vi "Read.vi"(8 "error in (no error)":errorcluster, 9 "Sample Rate [Hz]":dbl=1000.0 min=1000.0 max=8000000.0, 10 "Number of Samples":u32=1000, 11 "DI (N Samples) Ref In":T1) -> (0 "error out":errorcluster, 2 "Values":bool[][](array[boolean]), 3 "DI (N Samples) Ref Out":T1)   [LabVIEW 2021, in "DI Block.lvlib"]
doc: "Reads values from one or more digital input channels. Use this VI to read multiple samples for each channel at one time."
uses:
  <vilib>/myRIO/Instrument Drivers/Onboard IO/DI Block/DI Block.lvlib
  <vilib>/myRIO/Instrument Drivers/Onboard IO/DI Block/typedefs/DI Block Reference.ctl
  <vilib>/myRIO/Common/Instrument Driver Framework/Utilities/typedefs/myRIO Generic Hardware Reference.ctl
  <vilib>/myRIO/Common/Instrument Driver Framework/Utilities/typedefs/Hardware Version Enum.ctl
  <vilib>/myRIO/Common/Instrument Driver Framework/Utilities/typedefs/myRIO v1.0 Reference.ctl
  <vilib>/myRIO/Common/Instrument Driver Framework/Utilities/typedefs/Generic FPGA Reference.ctl
  <vilib>/myRIO/Common/Instrument Driver Framework/myRIO v1.0/DI Block/typedefs/DI Block Channels List.ctl
  <vilib>/myRIO/Common/Instrument Driver Framework/myRIO v1.0/DI Block/typedefs/DI Block Channels Enum.ctl
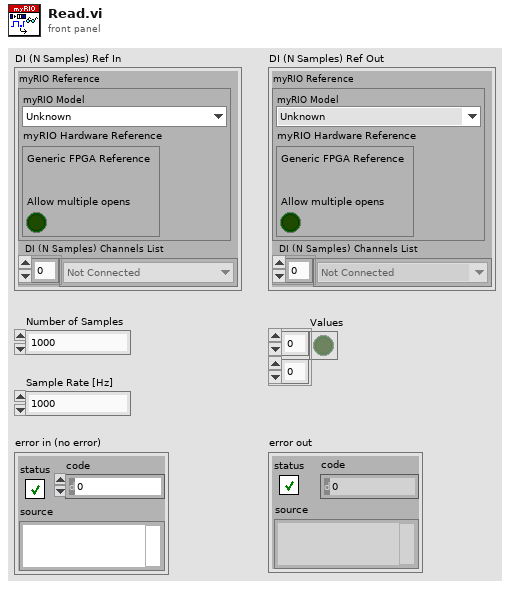
[diagram p1: front panel]
types:
  T1 = typedef "DI Block.lvlib/DI Block Reference.ctl" = cluster{"myRIO Reference":T2, "DI (N Samples) Channels List":T6}
  T2 = typedef "myRIO Generic Hardware Reference.ctl" = cluster{"myRIO Model":T3, "myRIO Hardware Reference":T4}
  T3 = typedef "Hardware Version Enum.ctl" = enum16{"Unknown", "myRIO-1900", "myRIO-1950", "roboRIO", "NI ELVIS RIO CM", "ELVIS III"}
  T4 = typedef "myRIO v1.0 Reference.ctl" = cluster{"Generic FPGA Reference":T5, "Allow multiple opens":bool}
  T5 = typedef "Generic FPGA Reference.ctl" = refnum<k20>
  T6 = typedef "DI Block Channels List.ctl" = T7[]
  T7 = typedef "DI Block Channels Enum.ctl" = enum16{"Not Connected", "A/DI0 (N Samples)", "A/DI1 (N Samples)", "A/DI2 (N Samples)", "A/DI3 (N Samples)", "A/DI4 (N Samples)", "A/DI5 (N Samples)", "A/DI6 (N Samples)", "A/DI7 (N Samples)", "A/DI8 (N Samples)", "A/DI9 (N Samples)", "A/DI10 (N Samples)", "A/DI11 (N Samples)", "A/DI12 (N Samples)", "A/DI13 (N Samples)", "A/DI14 (N Samples)", "A/DI15 (N Samples)", "A/DI16 (N Samples)", "A/DI17 (N Samples)", "A/DI18 (N Samples)", "A/DI19 (N Samples)", "B/DI0 (N Samples)", "B/DI1 (N Samples)", "B/DI2 (N Samples)", "B/DI3 (N Samples)", "B/DI4 (N Samples)", "B/DI5 (N Samples)", "B/DI6 (N Samples)", "B/DI7 (N Samples)", "B/DI8 (N Samples)", "B/DI9 (N Samples)", "B/DI10 (N Samples)", "B/DI11 (N Samples)", "B/DI12 (N Samples)", "B/DI13 (N Samples)", "B/DI14 (N Samples)", "B/DI15 (N Samples)", "B/DI16 (N Samples)", "B/DI17 (N Samples)", "B/DI18 (N Samples)", "B/DI19 (N Samples)"}
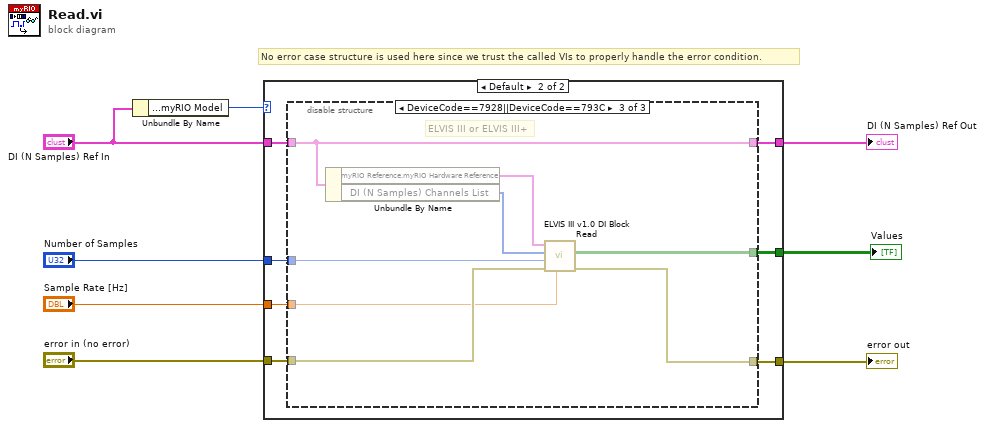
[diagram p0: block diagram]
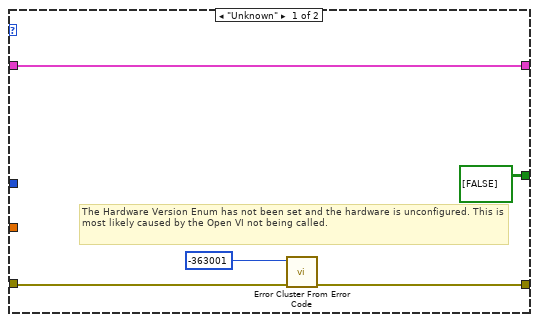
[diagram p2: hidden frame]
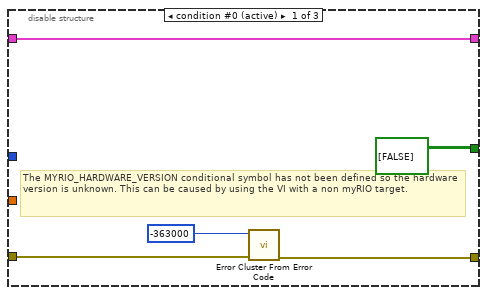
[diagram p3: hidden frame]
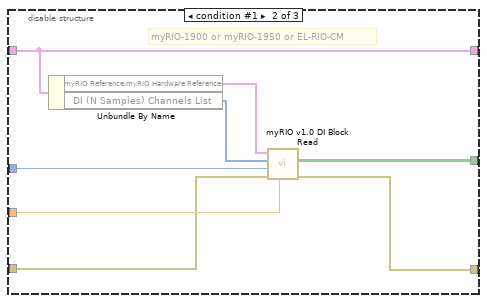
[diagram p4: hidden frame]
diagram:
  # "No error case structure is used here since we trust the called VIs to properly handle the error condition."
  n1 = Unbundle By Name("DI (N Samples) Ref In") -> ("myRIO Reference.myRIO Model"=w4:T3)
  n2 = case shown="Default" w4 {
    tunnel: [w11 w20] -> w5
    tunnel: "DI (N Samples) Ref In" -> [w10 w19]
    tunnel: "error in (no error)" -> [w12 w18]
    tunnel: [w10 w17] -> w6
    tunnel: "Sample Rate [Hz]" -> [_ w16]
    tunnel: "Number of Samples" -> [_ w15]
    tunnel: [bool[][] [[FALSE]] ("bool Value List") w14] -> w1
    frame "Unknown" {
      # "The Hardware Version Enum has not been set and the hardware is unconfigured. This is most likely caused by the Open VI not being called."
      n3 = call <vilib>:"Error Cluster From Error Code.vi"("error in (no error)"=w12, "error code (0)"=-363001) -> ("error out"=w11:errorcluster)  [unwired: 7 in]
    }
    frame Default {
      n4 = disable-structure shown="DeviceCode==7928||DeviceCode==793C" {
        disable-tunnel: w19 -> [w22 w26 w39]
        disable-tunnel: [w25 w32 w37] -> w20
        disable-tunnel: w18 -> [w23 w33 w36]
        disable-tunnel: [w22 w26 w39] -> w17
        disable-tunnel: w16 -> [_ w28 w35]
        disable-tunnel: w15 -> [_ w30 w34]
        disable-tunnel: [bool[][] [[FALSE]] ("bool Value List") w27 w38] -> w14
        frame condition #0 (active) {
          # "The MYRIO_HARDWARE_VERSION conditional symbol has not been defined so the hardware version is unknown. This can be caused by using the VI with a non myRIO target."
          n5 = call <vilib>:"Error Cluster From Error Code.vi"("error in (no error)"=w23, "error code (0)"=-363000) -> ("error out"=w25:errorcluster)  [unwired: 7 in]
        }
        frame condition #1 {
          # "myRIO-1900 or myRIO-1950 or EL-RIO-CM"
          n6 = Unbundle By Name(w26) -> ("myRIO Reference.myRIO Hardware Reference"=w31:T4, "DI (N Samples) Channels List"=w29:T6)
          n7 = call <vilib>:"myRIO v1.0 DI Block Read.vi"("DI FIFO Sample Rate (Hz)"=w28, "error in (no error)"=w33, "Number of Samples"=w30, "DI (N Samples) Channel List"=w29, "myRIO Ref In"=w31) -> ("error out"=w32:errorcluster, "bool Value List"=w27:bool[][])  [unwired: 4 in, 1 out]
        }
        frame condition #2 {
          # "ELVIS III or ELVIS III+"
          n8 = Unbundle By Name(w39) -> ("myRIO Reference.myRIO Hardware Reference"=w41:T4, "DI (N Samples) Channels List"=w40:T6)
          n9 = call <vilib>:"ELVIS III v1.0 DI Block Read.vi"("DI FIFO Sample Rate (Hz)"=w35, "error in (no error)"=w36, "Number of Samples"=w34, "DI (N Samples) Channel List"=w40, "myRIO Ref In"=w41) -> ("error out"=w37:errorcluster, "Data by Channel"=w38:bool[][])  [unwired: 4 in, 1 out]
        }
      }
    }
  }
  "DI (N Samples) Ref Out" <- w6
  "error out" <- w5
  "Values" <- w1
